vi "Calculate Formation Energies.vi"(4 "N Extrinsic Atoms":i32, 5 "Fermi (electron) energy (eV)":dbl=-2.0, 6 "# Extra Electrons":i32, 7 "Reference Elemental Bulk Energies":T4={"Energy of CdTe (eV/atom)"=-2.489625, "Energy of Cd (eV/atom)"=-0.9039318, "Energy of Te (eV/atom)"=-3.1404524}, 8 "N (Te,ideal - Te,defect)":i32, 9 "N (Cd,Ideal - Cd,Defect)":i32, 10 "Reference Pure Structure Energy":dbl=-358.247, 11 "Final Total Defect Energy (eV)":dbl=-2.48963) -> (2 "Formation Energy (Te-Rich)":dbl, 3 "Formation Energy (Cd-Rich)":dbl)   [LabVIEW 2010]
panel:
  in  "Missing Atoms Array":T1(array[cluster])
  in  "Chemical Potentials":T2(array[cluster])
  in  "System Cluster":T3={"Final Total Defect Energy (eV)"=-2.48963, "Reference Pure Structure Energy"=-358.247, "# Extra Electrons"=0, "Fermi (electron) energy (eV)"=-2.0}
  out "EForm 2":dbl
  out "Ed2 2":dbl
  out "Deltau 2":dbl
  out "uCd 2":dbl
  in  "uTe 2":dbl
  in  "Energy of Extrinsic X (eV/atom)":dbl
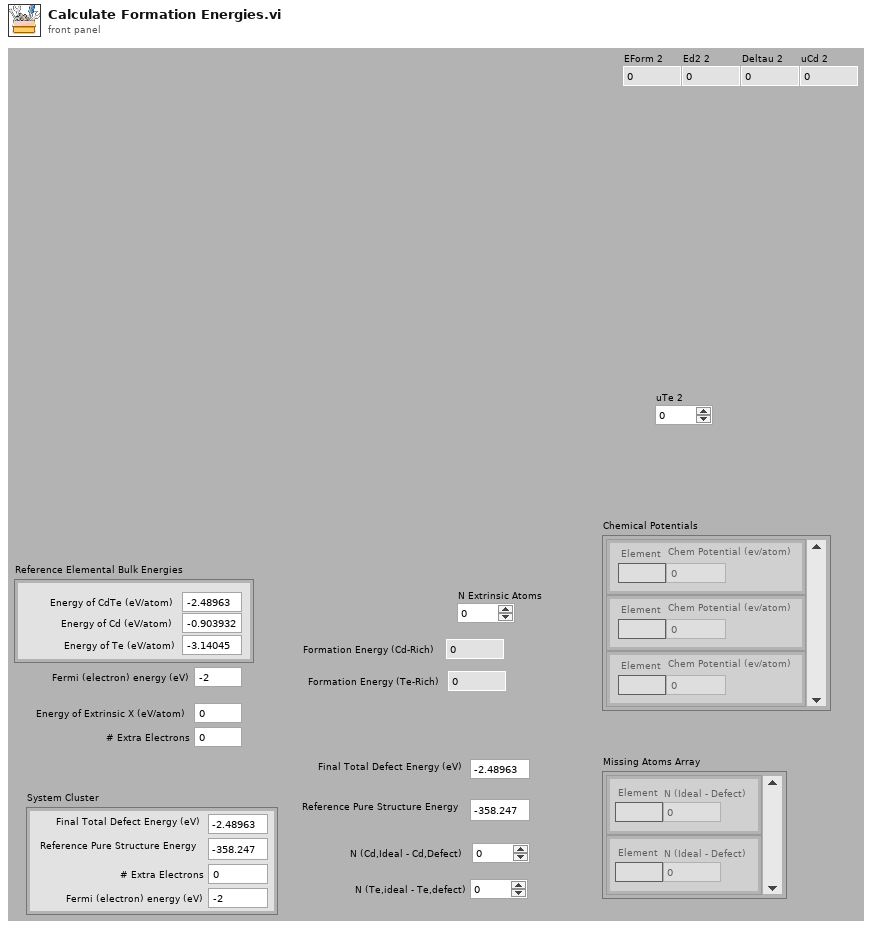
[diagram p1: front panel]
types:
  T1 = cluster{"Element":string, "N (Ideal - Defect)":i32}[]
  T2 = cluster{"Chem Potential (ev/atom)":dbl, "Element":string}[]
  T3 = cluster{"Final Total Defect Energy (eV)":dbl, "Reference Pure Structure Energy":dbl, "# Extra Electrons":i32, "Fermi (electron) energy (eV)":dbl}
  T4 = cluster{"Energy of CdTe (eV/atom)":dbl, "Energy of Cd (eV/atom)":dbl, "Energy of Te (eV/atom)":dbl}
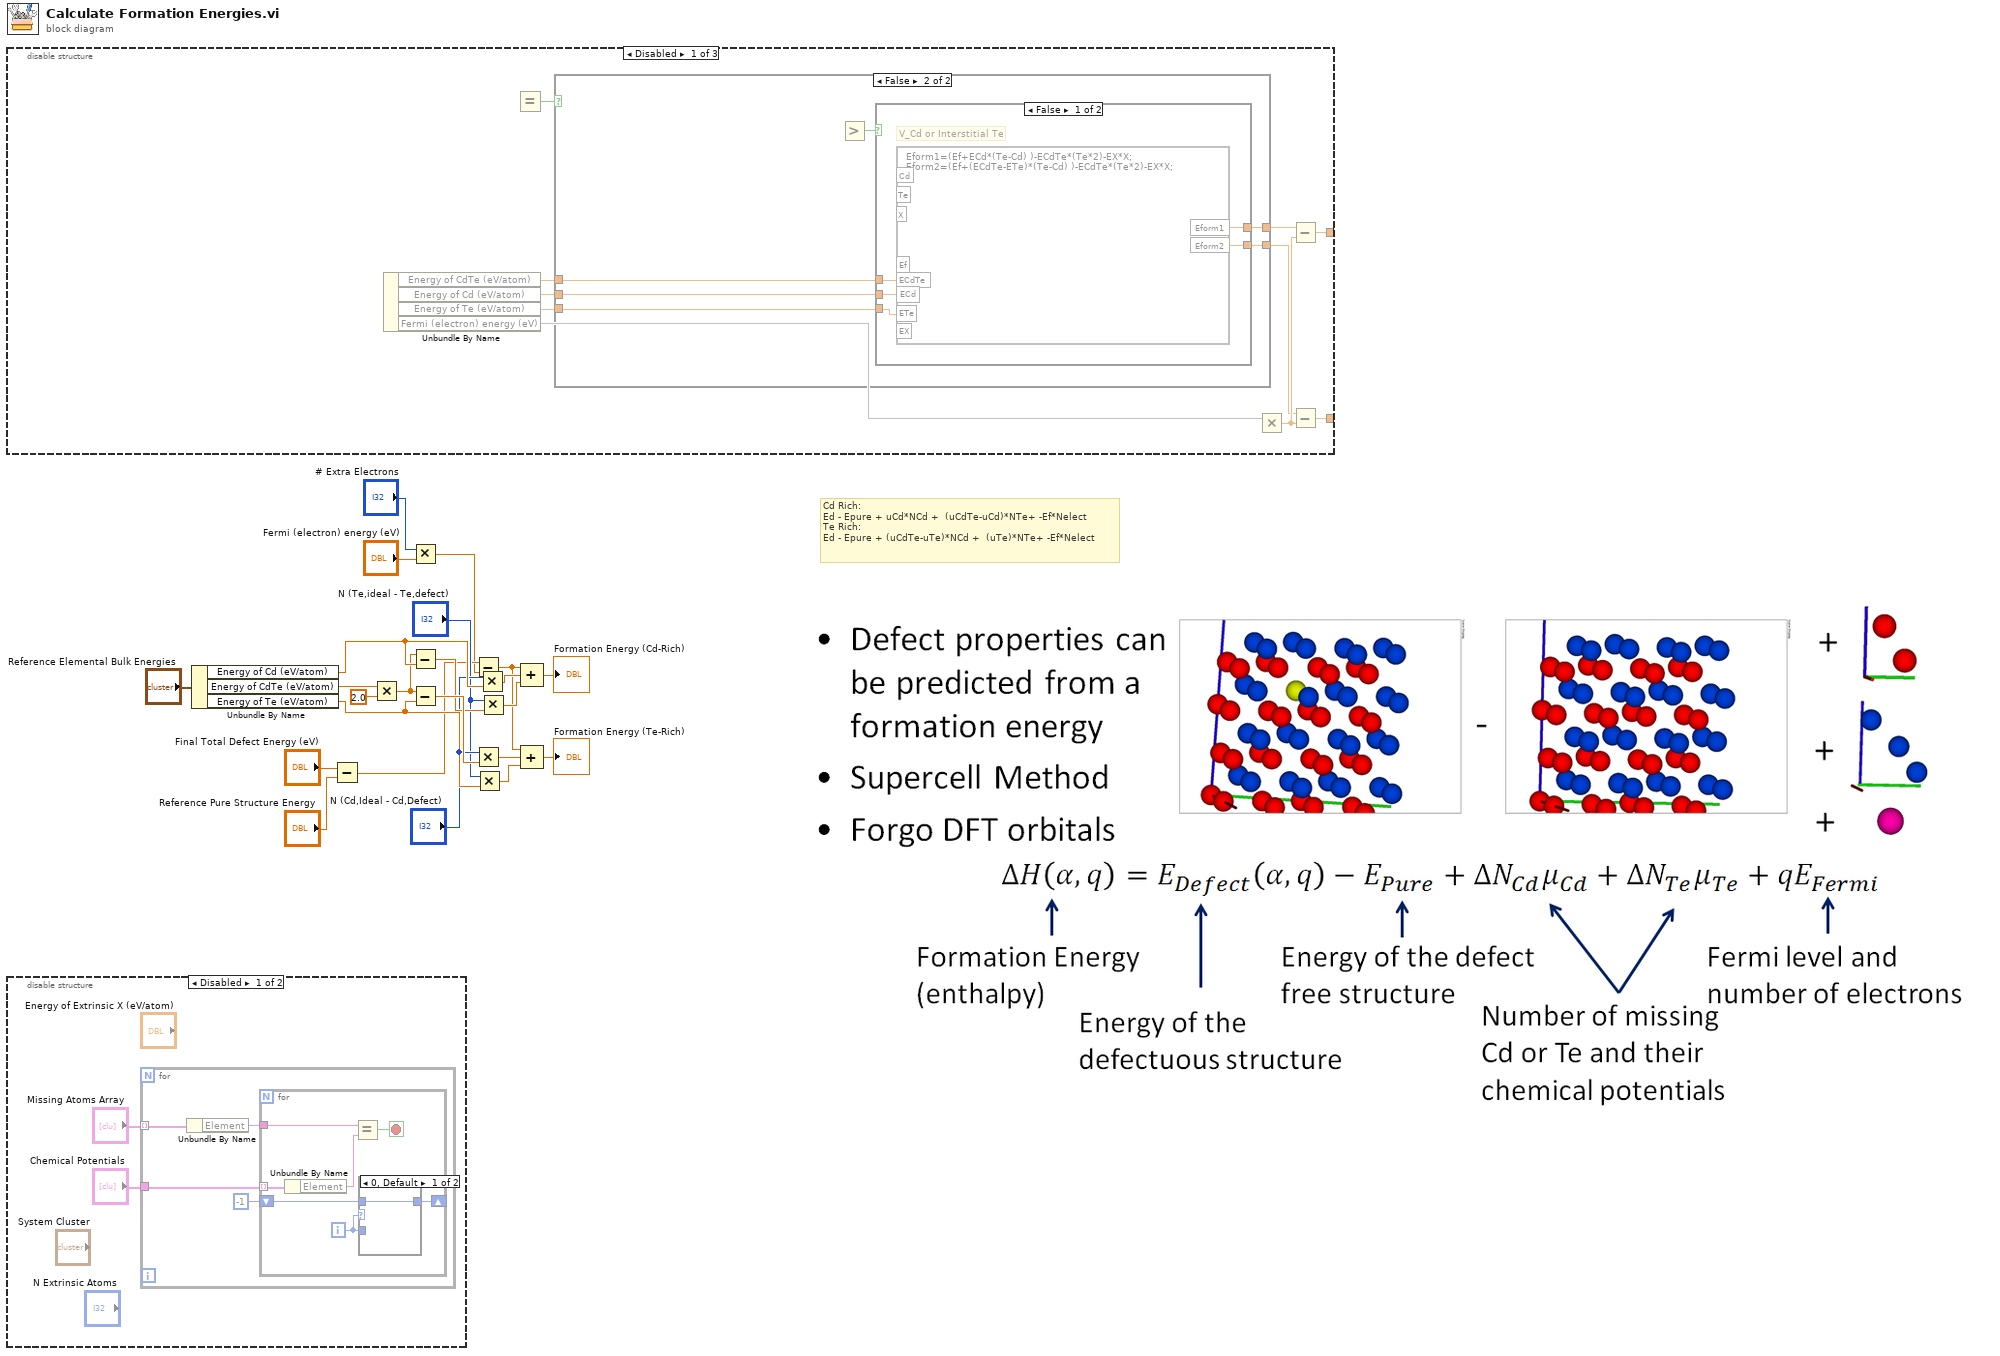
[diagram p0: block diagram]
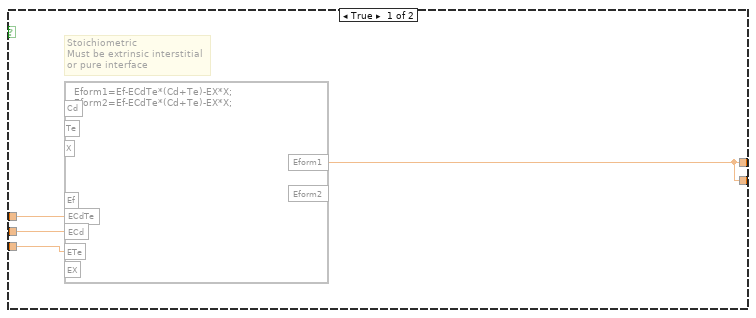
[diagram p4: hidden frame]
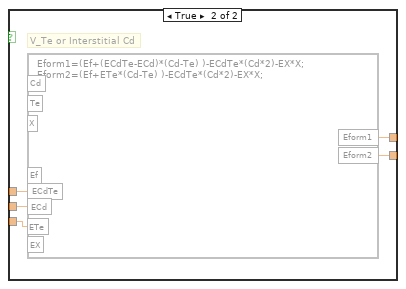
[diagram p5: hidden frame]
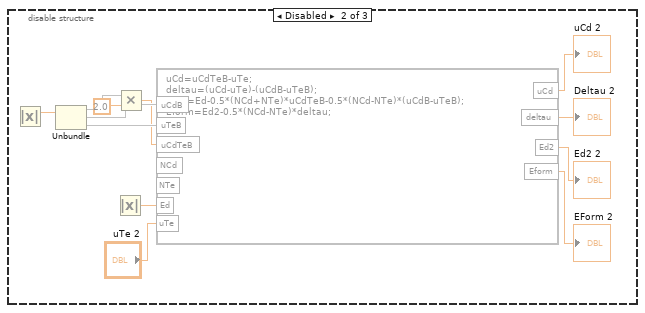
[diagram p6: hidden frame]
diagram:
  # "Cd Rich:\nEd - Epure + uCd*NCd +  (uCdTe-uCd)*NTe+ -Ef*Nelect\nTe Rich:\nEd - Epure + (uCdTe-uTe)*NCd +  (uTe)*NTe+ -Ef*Nelect"
  n1 = disable-structure shown="Disabled" {
    disable-tunnel: [w25 _ _] -> _
    disable-tunnel: [w24 _ _] -> _
    frame Disabled {
      n2 = Unbundle By Name() -> ("Energy of CdTe (eV/atom)"=w32:dbl, "Energy of Cd (eV/atom)"=w31:dbl, "Energy of Te (eV/atom)"=w30:dbl, "Fermi (electron) energy (eV)"=w29)  [unwired: 1 in]
      n3 = Equal?() -> (x = y?=w33:bool)  [unwired: 2 in]
      n4 = case shown="False" w33 {
        tunnel: w32 -> [w37 w43]
        tunnel: [w34 w39] -> w28
        tunnel: [w34 w38] -> w26
        tunnel: w31 -> [w36 w42]
        tunnel: w30 -> [w35 w41]
        frame True {
          # "Stoichiometric\nMust be extrinsic interstitial\nor pure interface"
          n5 = formula code="Eform1=Ef-ECdTe*(Cd+Te)-EX*X;\nEform2=Ef-ECdTe*(Cd+Te)-EX*X;"("ECdTe"=w37, "ECd"=w36, "ETe"=w35) -> ("Eform1"=w34:dbl)  [unwired: 5 in, 1 out]
        }
        frame False {
          n6 = Greater?() -> (0:w40:bool)  [unwired: 2 in]
          n7 = case shown="False" w40 {
            tunnel: w43 -> [w48 w53]
            tunnel: w42 -> [w47 w52]
            tunnel: w41 -> [w46 w51]
            tunnel: [w44 w49] -> w38
            tunnel: [w45 w50] -> w39
            frame False {
              # "V_Cd or Interstitial Te"
              n8 = formula code="Eform1=(Ef+ECd*(Te-Cd) )-ECdTe*(Te*2)-EX*X;\nEform2=(Ef+(ECdTe-ETe)*(Te-Cd) )-ECdTe*(Te*2)-EX*X;"("ECdTe"=w48, "ECd"=w47, "ETe"=w46) -> ("Eform1"=w45:dbl, "Eform2"=w44:dbl)  [unwired: 5 in]
            }
            frame True {
              # "V_Te or Interstitial Cd"
              n9 = formula code="Eform1=(Ef+(ECdTe-ECd)*(Cd-Te) )-ECdTe*(Cd*2)-EX*X;\nEform2=(Ef+ETe*(Cd-Te) )-ECdTe*(Cd*2)-EX*X;"("ECdTe"=w53, "ECd"=w52, "ETe"=w51) -> ("Eform1"=w50:dbl, "Eform2"=w49:dbl)  [unwired: 5 in]
            }
          }
        }
      }
      n10 = Multiply(x=w29) -> (x*y=w27:dbl)  [unwired: 1 in]
      n11 = Subtract(x=w28, y=w27) -> (x-y=w24:dbl)
      n12 = Subtract(x=w26, y=w27) -> (x-y=w25:dbl)
    }
    frame Disabled {
      n13 = Absolute Value() -> (abs(x)=w58:dbl)  [unwired: 1 in]
      n14 = Unbundle(w58) -> (w56, w65, w64)
      n15 = Absolute Value() -> (abs(x)=w57:dbl)  [unwired: 1 in]
      n16 = Multiply(x=w56, y=2.0) -> (x*y=w54:dbl)
      n17 = formula code="uCd=uCdTeB-uTe;\ndeltau=(uCd-uTe)-(uCdB-uTeB);\nEd2 =Ed-0.5*(NCd+NTe)*uCdTeB-0.5*(NCd-NTe)*(uCdB-uTeB);\nEform=Ed2-0.5*(NCd-NTe)*deltau;"("uCdB"=w65, "uTeB"=w64, "uCdTeB"=w54, "uTe"="uTe 2", "Ed"=w57) -> ("uCd"=→"uCd 2":dbl, "deltau"=→"Deltau 2":dbl, "Ed2"=→"Ed2 2":dbl, "Eform"=→"EForm 2":dbl)  [unwired: 2 in]
    }
    frame Enabled {
    }
  }
  n18 = disable-structure shown="Disabled" {
    frame Disabled {
      n19 = for {
        tunnel: "Missing Atoms Array" -> [w69] mode=indexing
        tunnel: "Chemical Potentials" -> [w71]
        n20 = Unbundle By Name(w69) -> ("Element"=w68:string)
        n21 = for {
          tunnel: w71 -> [w78] mode=indexing
          shift-right: [w75] -> _
          shift-left: -1 -> [w74]
          tunnel: w68 -> [w73]
          i -> [w72]
          stop <- w76 stop-if-true
          n22 = Unbundle By Name(w78) -> ("Element"=w77:string)
          n23 = Equal?(x=w73, y=w77) -> (x = y?=w76:bool)
          n24 = case shown="0, Default" w72 {
            tunnel: [w79 w80] -> w75
            tunnel: w72 -> [_ w80]
            tunnel: w74 -> [w79 _]
            frame 0, Default {
            }
            frame 1 {
            }
          }
        }
      }
    }
    frame Enabled {
    }
  }
  n25 = Unbundle By Name("Reference Elemental Bulk Energies") -> ("Energy of Cd (eV/atom)"=w10:dbl, "Energy of CdTe (eV/atom)"=w11:dbl, "Energy of Te (eV/atom)"=w8:dbl)
  n26 = Subtract(x="Final Total Defect Energy (eV)", y="Reference Pure Structure Energy") -> (x-y=w4:dbl)
  n27 = Multiply(x=w11, y=2.0) -> (x*y=w1:dbl)
  n28 = Multiply(x="# Extra Electrons", y="Fermi (electron) energy (eV)") -> (x*y=w3:dbl)
  n29 = Subtract(x=w1, y=w10) -> (x-y=w9:dbl)
  n30 = Subtract(x=w1, y=w8) -> (x-y=w12:dbl)
  n31 = Subtract(x=w4, y=w3) -> (x-y=w2:dbl)
  n32 = Multiply(x="N (Cd,Ideal - Cd,Defect)", y=w12) -> (x*y=w16:dbl)
  n33 = Multiply(x="N (Te,ideal - Te,defect)", y=w8) -> (x*y=w14:dbl)
  n34 = Multiply(x="N (Cd,Ideal - Cd,Defect)", y=w10) -> (x*y=w17:dbl)
  n35 = Multiply(x="N (Te,ideal - Te,defect)", y=w9) -> (x*y=w15:dbl)
  n36 = Compound Arithmetic op=ADD(w2, w17, w15) -> (→"Formation Energy (Cd-Rich)":dbl)
  n37 = Compound Arithmetic op=ADD(w2, w16, w14) -> (→"Formation Energy (Te-Rich)":dbl)
